vi "RAZ DTC J1 AUTO.vi"(8 "errin":errorcluster, 11 "Boitier J1 auto":refnum<visa-resource-name>) -> (0 "sortie d'erreur":errorcluster caption="errout", 3 "=no DTC ?":bool)   [LabVIEW 2020]
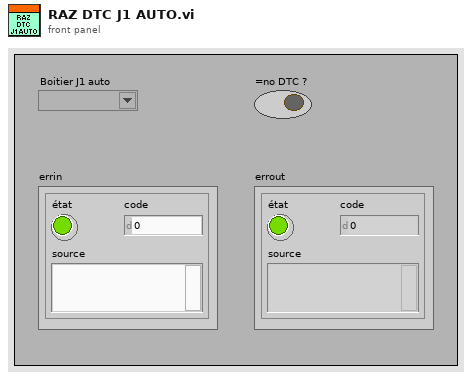
[diagram p1: front panel]
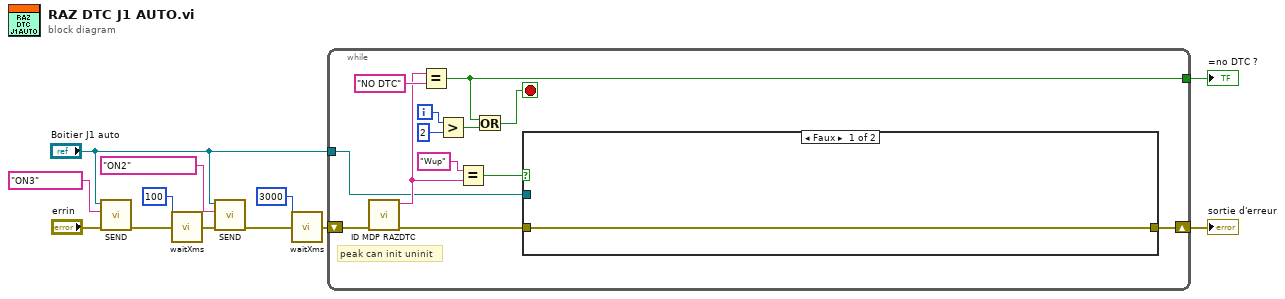
[diagram p0: block diagram]
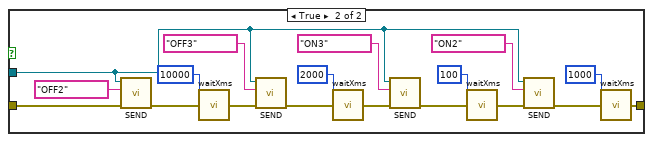
[diagram p2: hidden frame]
diagram:
  n1 = call "SEND.vi"("errin"="errin", "chaîne"="ON3" ("CMD"), "visa in"="Boitier J1 auto") -> ("errout"=w3:errorcluster)  [unwired: 6 in, 2 out]
  n2 = call "waitXms.vi"("attente (ms)"=u32 100, "errin"=w3) -> ("errout"=w5:errorcluster)  [unwired: 13 in]
  n3 = call "SEND.vi"("errin"=w5, "chaîne"="ON2" ("CMD"), "visa in"="Boitier J1 auto") -> ("errout"=w7:errorcluster)  [unwired: 6 in, 2 out]
  n4 = call "waitXms.vi"("attente (ms)"=u32 3000, "errin"=w7) -> ("errout"=w9:errorcluster)  [unwired: 13 in]
  n5 = while {
    shift-right: [w15] -> w1
    shift-left: w9 -> [w25]
    tunnel: [w17] -> w2
    tunnel: "Boitier J1 auto" -> [w13]
    i -> [w22]
    stop <- w18 stop-if-true
    # "peak can init uninit"
    n6 = call "ID MDP RAZDTC.vi"("errin"=w25) -> ("errout"=w16:errorcluster, "MSG"=w20:string)  [unwired: 7 in, 2 out]
    n7 = Equal?(x=w20, y="NO DTC") -> (x = y?=w17:bool)
    n8 = Greater?(x=w22, y=2) -> (0:w19:bool)
    n9 = Equal?(x="Wup", y=w20) -> (x = y?=w14:bool)
    n10 = Or(x=w17, y=w19) -> (x .or. y?=w18:bool)
    n11 = case shown="Faux" w14 {
      tunnel: w16 -> [w26 w44]
      tunnel: [w26 w31] -> w15
      tunnel: w13 -> [_ w30]
      frame False {
      }
      frame True {
        n12 = call "SEND.vi"("errin"=w44, "chaîne"="OFF2" ("CMD"), "visa in"=w30) -> ("errout"=w42:errorcluster)  [unwired: 6 in, 2 out]
        n13 = call "waitXms.vi"("attente (ms)"=u32 10000, "errin"=w42) -> ("errout"=w40:errorcluster)  [unwired: 13 in]
        n14 = call "SEND.vi"("errin"=w40, "chaîne"="OFF3" ("CMD"), "visa in"=w30) -> ("errout"=w38:errorcluster)  [unwired: 6 in, 2 out]
        n15 = call "waitXms.vi"("attente (ms)"=u32 2000, "errin"=w38) -> ("errout"=w32:errorcluster)  [unwired: 13 in]
        n16 = call "SEND.vi"("errin"=w32, "chaîne"="ON3" ("CMD"), "visa in"=w30) -> ("errout"=w37:errorcluster)  [unwired: 6 in, 2 out]
        n17 = call "waitXms.vi"("attente (ms)"=u32 100, "errin"=w37) -> ("errout"=w35:errorcluster)  [unwired: 13 in]
        n18 = call "SEND.vi"("errin"=w35, "chaîne"="ON2" ("CMD"), "visa in"=w30) -> ("errout"=w33:errorcluster)  [unwired: 6 in, 2 out]
        n19 = call "waitXms.vi"("attente (ms)"=u32 1000, "errin"=w33) -> ("errout"=w31:errorcluster)  [unwired: 13 in]
      }
    }
  }
  "=no DTC ?" <- w2
  "sortie d'erreur" <- w1
